vi "NXTSumoEyes-Remote.vi"() -> ()   [LabVIEW 2009]
uses:
  <vilib>/NXT/Subs/LVHSConnector.ctl
  <vilib>/NXT/Block Support/NXT_InputPort.ctl
panel:
  in  "Select Range":u16(ring)=6 items=["short"=5, "long"=6]
  in  "Ring 2":u16(ring)=6 items=["short"=5, "long"=6]
  in  "?":bool=TRUE
  in  "Input Port":T1 items=["Port 1", "Port 2", "Port 3", "Port 4"]
  in  "NXT":T2={"error"={"status"=FALSE, "code"=0, "source"=""}, "address"="", "NXT #"=-1, "Show Error"=TRUE}
  out "NXT dup":T2={"error"={"status"=FALSE, "code"=0, "source"=""}, "address"="", "NXT #"=-1, "Show Error"=TRUE}
  # "mindsensors.com\nCopyright (c) 2009 by mindsensors.com\nEmail: info (<at>) mindsensors (<dot>) com\n\nThis program is free software. You can redistribute it and/or modify\nit under the terms of the GNU General Public License as published by\nthe Free Software Foundation; version 3 of the License.\nRead the license at: http://www.gnu.org/licenses/gpl.txt"
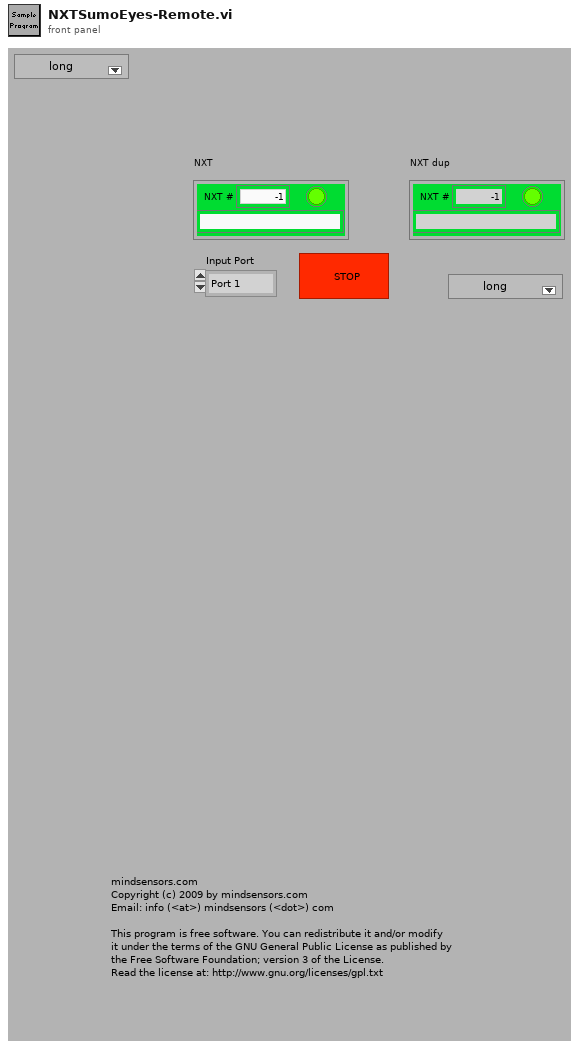
[diagram p1: front panel]
types:
  T1 = typedef "NXT_InputPort.ctl" = u8
  T2 = typedef "LVHSConnector.ctl" = cluster{"error":errorcluster, "address":string, "NXT #":i32, "Show Error":bool}
  T3 = cluster{"Start X":i16, "Start  Y":i16, "Width":i16, "Height":i16}
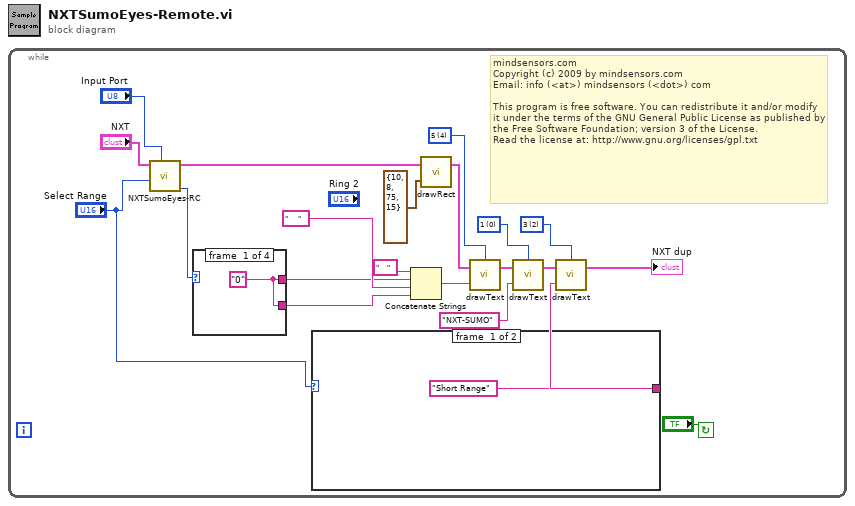
[diagram p0: block diagram]
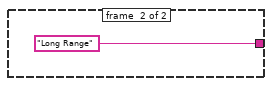
[diagram p2: hidden frame]
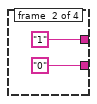
[diagram p3: hidden frame]
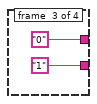
[diagram p4: hidden frame]
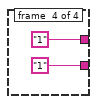
[diagram p5: hidden frame]
diagram:
  n1 = while {
    stop <- "?" continue-if-true
    w5 = i16 2 items=["1", "2", "3", "4", "5", "6", "7", "8"] ("Line")
    w10 = i16 0 items=["1", "2", "3", "4", "5", "6", "7", "8"] ("Line")
    w16 = i16 4 items=["1", "2", "3", "4", "5", "6", "7", "8"] ("Line")
    # "mindsensors.com\nCopyright (c) 2009 by mindsensors.com\nEmail: info (<at>) mindsensors (<dot>) com\n\nThis program is free software. You can redistribute it and/or modify\nit under the terms of the GNU General Public License as published by\nthe Free Software Foundation; version 3 of the License.\nRead the license at: http://www.gnu.org/licenses/gpl.txt"
    n2 = call "NXTSumoEyes-RC.vi"("Input Port"="Input Port", "Select Range"="Select Range", "NXT"="NXT") -> ("What Zone?"=w2:u8, "NXT dup"=w17:T2)  [unwired: 6 in, 1 out]
    n3 = case shown="0, Default" w2 {
      tunnel: [w24 "1" "0" "1"] -> w8
      tunnel: [w24 "0" "1" "1"] -> w7
      frame #0 {
        w24 = "0"
      }
      frame #1 {
      }
      frame #2 {
      }
      frame #3 {
      }
    }
    n4 = case shown="1" "Select Range" {
      tunnel: ["Short Range" "Long Range"] -> w3
      frame #0 {
      }
      frame #1 {
      }
    }
    n5 = Concatenate Strings("    " ("string"), w8, "     " ("string"), w7) -> (w13:string)
    n6 = call <vilib>:"drawRect.vi"("Rect Parameters"=T3 {"Start X"=10, "Start  Y"=8, "Width"=75, "Height"=15}, "NXT"=w17) -> ("NXT"=w12:T2)  [unwired: 2 in]
    n7 = call <vilib>:"drawText.vi"("Text"=w13, "NXT"=w12, "Line"=w16) -> ("NXT"=w11:T2)  [unwired: 1 in]
    n8 = call <vilib>:"drawText.vi"("Text"="NXT-SUMO", "NXT"=w11, "Line"=w10) -> ("NXT"=w6:T2)  [unwired: 1 in]
    n9 = call <vilib>:"drawText.vi"("Text"=w3, "NXT"=w6, "Line"=w5) -> ("NXT"=→"NXT dup":T2)  [unwired: 1 in]
  }
